vi "Delete Diagram SubVIs.vi"(8 "error in (no error)":errorcluster, 11 "Diagram in":refnum<vi>) -> (0 "error out":errorcluster, 3 "Diagram out":refnum<vi>)   [LabVIEW 2019, in "gRPC Scripting Tools.lvlib"]
uses:
  gRPC Scripting Tools.lvlib
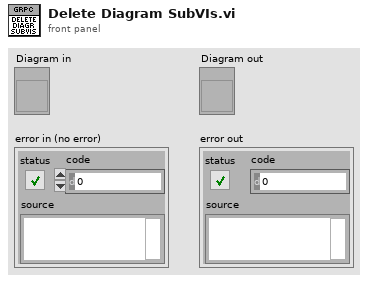
[diagram p1: front panel]
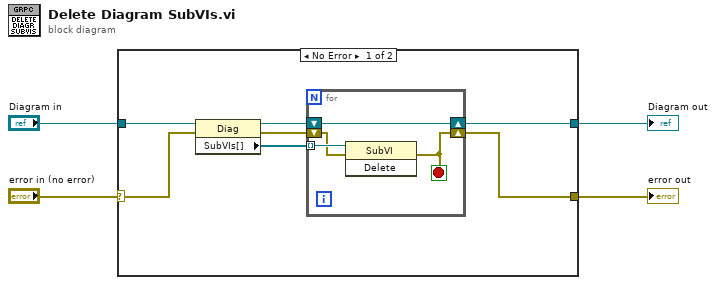
[diagram p0: block diagram]
diagram:
  n1 = case shown="No Error" "error in (no error)" {
    selector: "error in (no error)" -> [w5 w16]
    tunnel: [w11 w17] -> w4
    tunnel: [w10 w16] -> w3
    tunnel: "Diagram in" -> [w6 w17]
    frame No Error {
      n2 = property class="Diag"(reference=w6, error in=w5) -> (reference out=w9:refnum<vi>, error out=w8:errorcluster, "SubVIs[]"=w7:refnum<vi>[])
      n3 = for {
        tunnel: w7 -> [w15] mode=indexing
        shift-right: [w12] -> w10
        shift-left: w8 -> [w13]
        shift-right: [w14] -> w11
        shift-left: w9 -> [w14]
        stop <- w12 stop-if-true
        n4 = invoke class="SubVI" method="Delete"(reference=w15, error in=w13) -> (error out=w12:errorcluster)  [unwired: 1 in, 2 out]
      }
    }
    frame Error {
    }
  }
  "Diagram out" <- w4
  "error out" <- w3
